vi "ConfigureAsyncCore.vi"(8 "error in (no error)":errorcluster, 11 "MicronGRPCClient in":refnum<class "MicronGRPCClient.lvclass">) -> (0 "error out":errorcluster, 3 "MicronGRPCClient out":refnum<class "MicronGRPCClient.lvclass">)   [LabVIEW 2019, in "MicronGRPCClient.lvclass"]
uses:
  MicronGRPCClient.lvclass
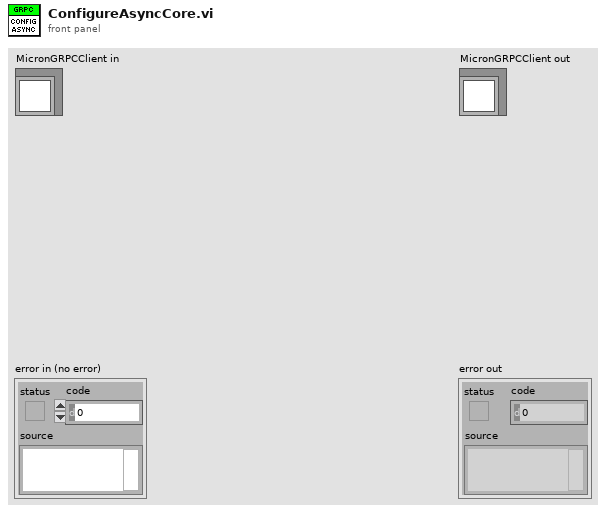
[diagram p1: front panel]
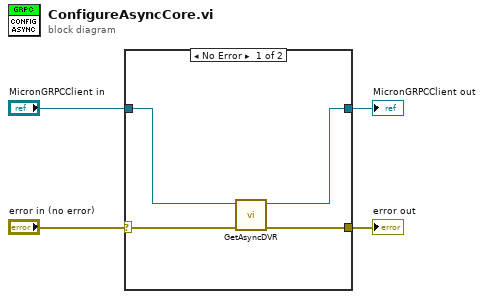
[diagram p0: block diagram]
diagram:
  n1 = case shown="No Error" "error in (no error)" {
    selector: "error in (no error)" -> [w8 w10]
    tunnel: [w7 w10] -> w3
    tunnel: [w5 w9] -> w1
    tunnel: "MicronGRPCClient in" -> [w6 w9]
    frame No Error {
      n2 = call-dynamic "GetAsyncDVR.vi"("error in (no error)"=w8, "MicronGRPCClient in"=w6) -> ("error out"=w7:errorcluster, "MicronGRPCClient out"=w5:refnum<class "MicronGRPCClient.lvclass">)  [unwired: 7 in, 1 out]
    }
    frame Error {
    }
  }
  "error out" <- w3
  "MicronGRPCClient out" <- w1
